vi "Test CSPD.vi"() -> ()   [LabVIEW 2020]
uses:
  epl-vi-lib/Signal Synthesis VIs/4th Generation/Classes/Level/LevelUnits.ctl
  epl-vi-lib/Signal Synthesis VIs/4th Generation/Classes/Filter/Shape.ctl
  epl-vi-lib/Signal Synthesis VIs/4th Generation/Classes/Filter/Units.ctl
  epl-vi-lib/Signal Synthesis VIs/4th Generation/Classes/Filter/Class.ctl
  epl-vi-lib/Signal Synthesis VIs/4th Generation/Classes/Level/Level.lvclass/Level.ctl
  epl-vi-lib/Signal Synthesis VIs/4th Generation/Classes/Filter/Filter.lvclass/Filter.ctl
  epl-vi-lib/Signal Synthesis VIs/4th Generation/Classes/Channel/Channel.lvclass/Channel.ctl
  epl-vi-lib/Signal Synthesis VIs/4th Generation/Classes/Waveforms/Noise/Noise.lvclass/Noise.ctl
  3524247a-8ae7-46d9-b71a-c66d4844bc9f.vi
  515af87e-e52d-4374-9cab-fcd7ae8fdb32.vi
  d0648034-2dec-4c64-9990-624be246044c.vi
  <vilib>/Analysis/baseanly.llb/Mean (DBL).vi
  6fae71c9-6d50-4778-9b27-4de804f51e00.vi
  <vilib>/Analysis/2dsp.llb/Cross Power (DBL).vi
  726719d0-53ab-4cde-bbae-18d33152857b.vi
  2604dc13-bcb2-40bf-816d-3a5cc3b7061b.vi
  1f3778f6-1701-4067-84f0-78bcc854d358.vi
  98786886-4506-48be-a372-97a999c07828.vi
  42c39028-ae27-4509-9454-5f7b85e5a68c.vi
  b4e7675a-24cb-4713-9642-d50581707a3a.vi
  epl-vi-lib/Signal Synthesis VIs/4th Generation/Classes/Waveforms/Noise/Write Weights.vi
  epl-vi-lib/Signal Synthesis VIs/4th Generation/Classes/Level/Write Units.vi
  epl-vi-lib/Signal Synthesis VIs/4th Generation/Classes/Level/Write Level.vi
  epl-vi-lib/Signal Synthesis VIs/4th Generation/Classes/Filter/Write Type.vi
  epl-vi-lib/Signal Synthesis VIs/4th Generation/Classes/Filter/Write Units.vi
  epl-vi-lib/Signal Synthesis VIs/4th Generation/Classes/Filter/Write BW (kHz).vi
  epl-vi-lib/Signal Synthesis VIs/4th Generation/Classes/Filter/Write CF (kHz).vi
  epl-vi-lib/Signal Synthesis VIs/4th Generation/Classes/Filter/Write Class.vi
  epl-vi-lib/Signal Synthesis VIs/4th Generation/Classes/Channel/Write Waveform.vi
  epl-vi-lib/Signal Synthesis VIs/4th Generation/Classes/Channel/Write Level.vi
  epl-vi-lib/Signal Synthesis VIs/4th Generation/Classes/Channel/Write Destination.vi
  epl-vi-lib/Signal Synthesis VIs/4th Generation/Classes/Channel/Write Filter.vi
  epl-vi-lib/Signal Synthesis VIs/4th Generation/Classes/Waveforms/Noise/Noise.lvclass
  D:/Development/epl-vi-lib/Signal Synthesis VIs/4th Generation/Classes/Waveforms/Waveform/Waveform.lvclass
  epl-vi-lib/Utility VIs/Math VIs/FFT x(t) to dB,Degrees (1D).vi
  epl-vi-lib/Signal Synthesis VIs/4th Generation/Classes/Channel/Channel.lvclass
  epl-vi-lib/Signal Synthesis VIs/4th Generation/Classes/Level/Level.lvclass
  epl-vi-lib/Signal Synthesis VIs/4th Generation/Classes/SignalManager/SignalManager.lvclass
  epl-vi-lib/Signal Synthesis VIs/4th Generation/Classes/Filter/Filter.lvclass
  <vilib>/Analysis/NI_AALPro.lvlib
  <vilib>/Analysis/NI_AALBase.lvlib
panel:
  out "Pcs 3":dbl
  out "mean":dbl format="%.7f"
  out "Pcs 2":dbl
  out "Pcs":dbl
  out "Px":dbl
  out "XY Graph":T1(graph)
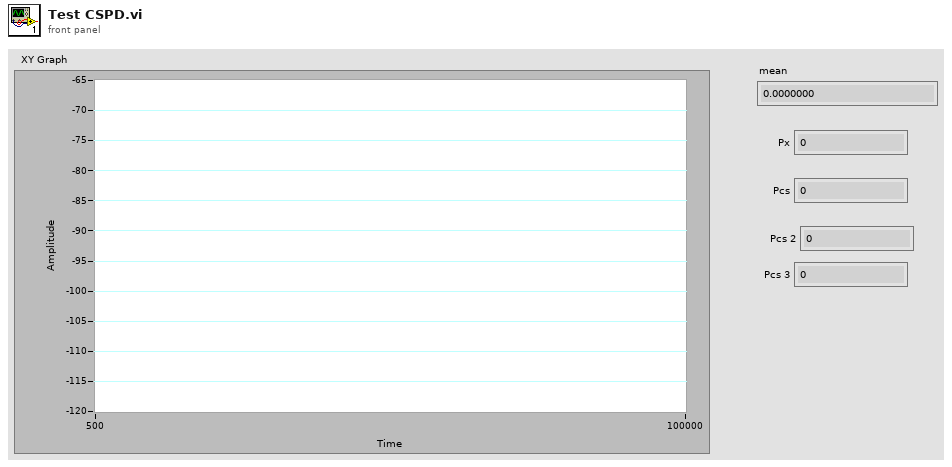
[diagram p1: front panel]
types:
  T1 = cluster{"Freq (Hz)":dbl[], "+Freq. Mag of FFT (dB rms)":dbl[]}[]
  T2 = typedef "Filter.lvclass/Class.ctl" = enum16{"Elliptic", "Butterworth", "Brickwall"}
  T3 = typedef "Filter.lvclass/Units.ctl" = enum16{"Linear", "Octaves", "Min-Max"}
  T4 = typedef "Filter.lvclass/Shape.ctl" = enum16{"OFF", "Lowpass", "Highpass", "Bandpass", "Bandstop"}
  T5 = typedef "Level.lvclass/LevelUnits.ctl" = enum16{"dB atten", "dB SPL", "dB Vrms", "Volts", "dB mW", "mW", "dB HL", "dB SL"}
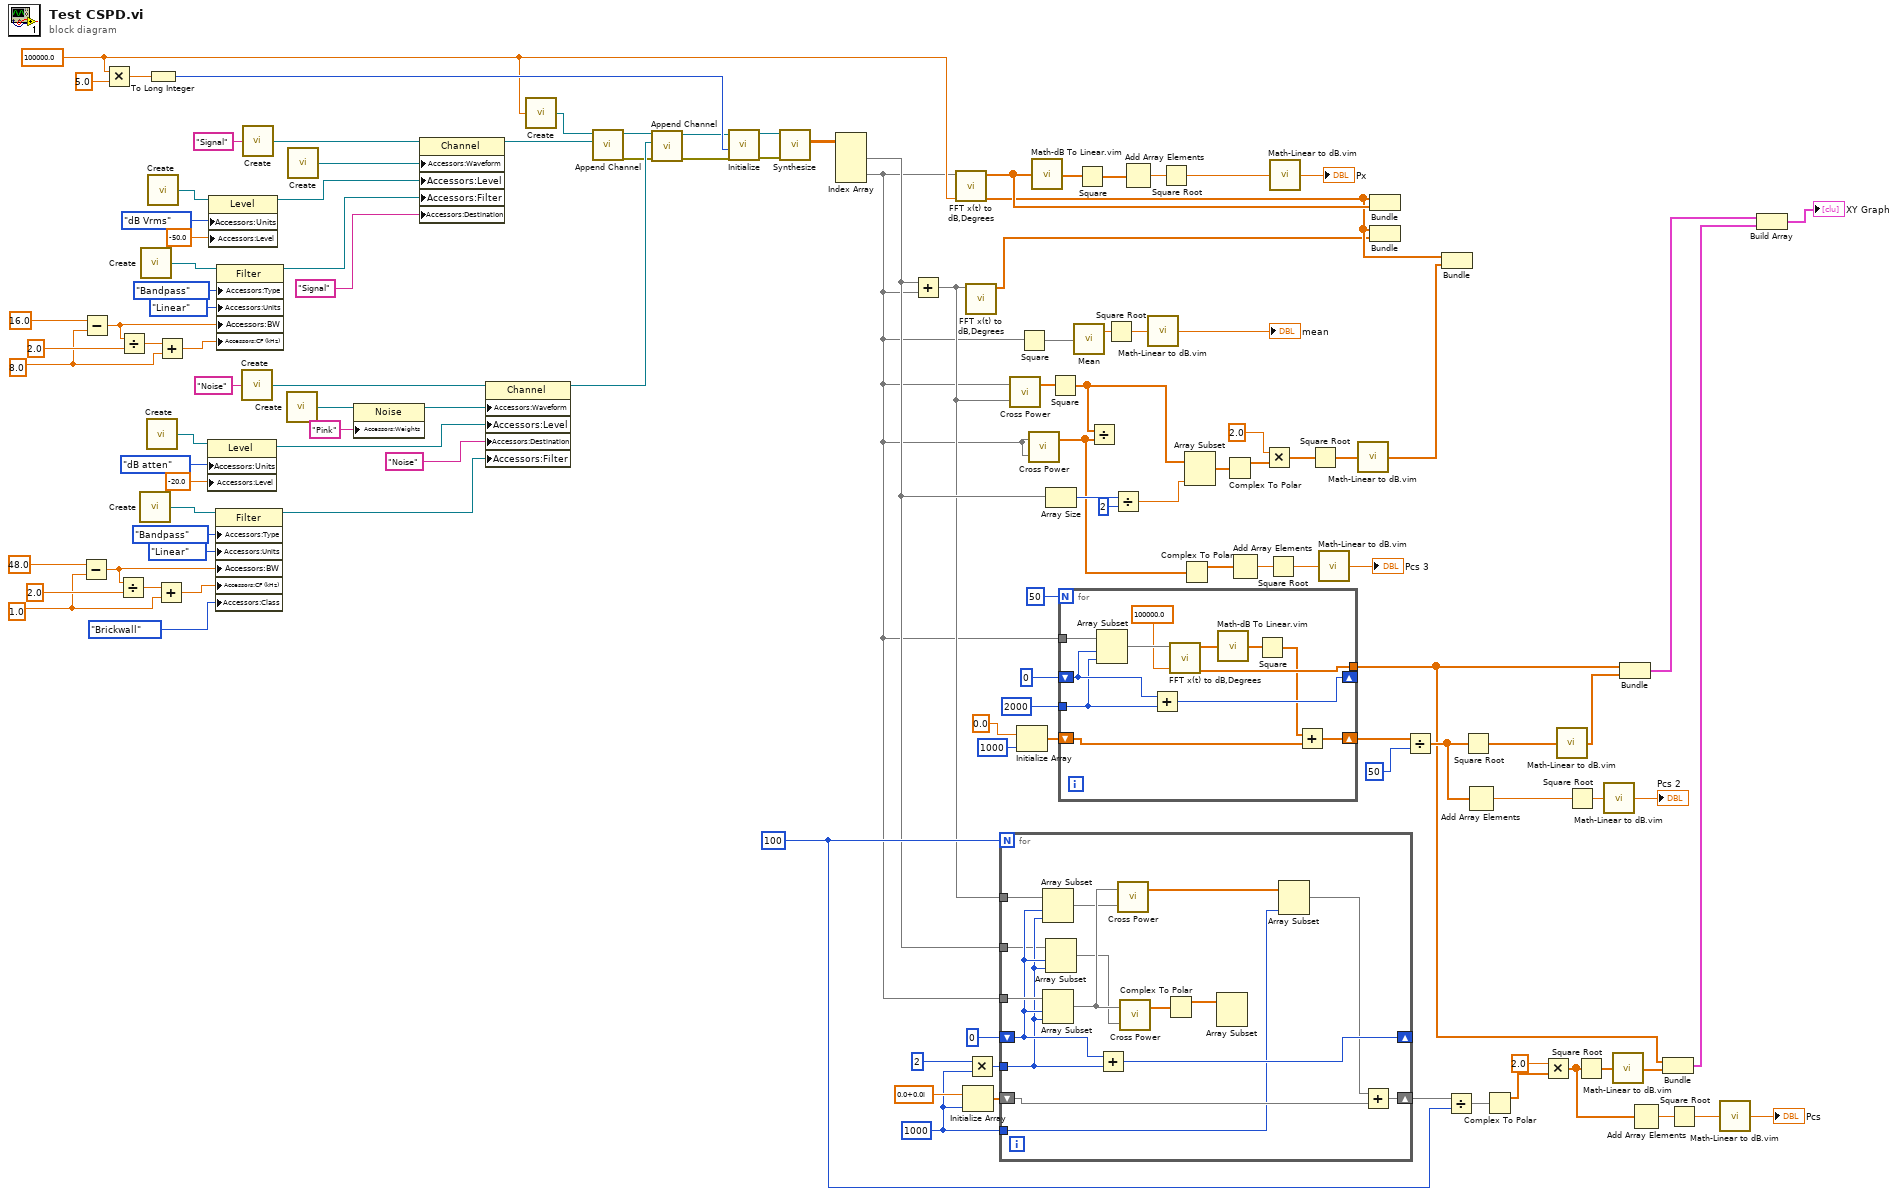
[diagram p0: block diagram]
diagram:
  w31 = 1000 ("dimension size")
  w29 = 100
  w81 = 1.0 ("High cutoff (kHz)")
  w97 = 100000.0 ("Fs (Hz)")
  w101 = 8.0 ("High cutoff (kHz)")
  n1 = Subtract(x=48.0 ("High cutoff (kHz)"), y=w81) -> (x-y=w85:dbl)
  n2 = Subtract(x=16.0 ("High cutoff (kHz)"), y=w101) -> (x-y=w108:dbl)
  n3 = Multiply(x=w97, y=5.0) -> (x*y=w99:dbl)
  n4 = Divide(x=w85, y=2.0) -> (x/y=w95:dbl)
  n5 = Divide(x=w108, y=2.0) -> (x/y=w118:dbl)
  n6 = call "Create.vi"() -> ("Filter"=w88:refnum<class "Filter.lvclass">)  [unwired: 15 in]
  n7 = call "Create.vi"() -> ("Filter"=w111:refnum<class "Filter.lvclass">)  [unwired: 15 in]
  n8 = call "Create.vi"() -> ("Level"=w92:refnum<class "Level.lvclass">)  [unwired: 15 in]
  n9 = To Long Integer(number=w99) -> (32bit integer=w98:i32)
  n10 = call "Create.vi"() -> ("Level"=w115:refnum<class "Level.lvclass">)  [unwired: 15 in]
  n11 = Add(x=w95, y=w81) -> (x+y=w84:dbl)
  n12 = Add(x=w118, y=w101) -> (x+y=w107:dbl)
  n13 = property class="Level"(reference=w92, "Accessors:Units"=LevelUnits."dB atten" ("Units"), "Accessors:Level"=-20.0 ("Level")) -> (reference out=w89:refnum<class "Level.lvclass">)  [unwired: 1 in, 1 out]
  n14 = property class="Level"(reference=w115, "Accessors:Units"=LevelUnits."dB Vrms" ("Units"), "Accessors:Level"=-50.0 ("Level")) -> (reference out=w112:refnum<class "Level.lvclass">)  [unwired: 1 in, 1 out]
  n15 = property class="Filter"(reference=w88, "Accessors:Type"=Shape."Bandpass" ("Type"), "Accessors:Units"=Units."Linear" ("Units"), "Accessors:BW"=w85, "Accessors:CF (kHz)"=w84, "Accessors:Class"=Class."Brickwall" ("Class")) -> (reference out=w9:refnum<class "Filter.lvclass">)  [unwired: 1 in, 1 out]
  n16 = property class="Filter"(reference=w111, "Accessors:Type"=Shape."Bandpass" ("Type"), "Accessors:Units"=Units."Linear" ("Units"), "Accessors:BW"=w108, "Accessors:CF (kHz)"=w107) -> (reference out=w106:refnum<class "Filter.lvclass">)  [unwired: 1 in, 1 out]
  n17 = call "Create.vi"("Name"="Noise") -> ("Channel"=w93:refnum<class "Channel.lvclass">)  [unwired: 14 in]
  n18 = call "Create.vi"("Name"="Signal") -> ("Channel"=w116:refnum<class "Channel.lvclass">)  [unwired: 14 in]
  n19 = call "Create.vi"() -> ("Noise"=w80:refnum<class "Noise.lvclass">)  [unwired: 15 in]
  n20 = call "Create.vi"() -> ("Noise"=w10:refnum<class "Noise.lvclass">)  [unwired: 15 in]
  n21 = property class="Noise"(reference=w80, "Accessors:Weights"="Pink" ("Weights")) -> (reference out=w79:refnum<class "Noise.lvclass">)  [unwired: 1 in, 1 out]
  n22 = property class="Channel"(reference=w116, "Accessors:Waveform"=w10, "Accessors:Level"=w112, "Accessors:Filter"=w106, "Accessors:Destination"="Signal") -> (reference out=w104:refnum<class "Channel.lvclass">)  [unwired: 1 in, 1 out]
  n23 = property class="Channel"(reference=w93, "Accessors:Waveform"=w79, "Accessors:Level"=w89, "Accessors:Destination"="Noise", "Accessors:Filter"=w9) -> (reference out=w76:refnum<class "Channel.lvclass">)  [unwired: 1 in, 1 out]
  n24 = call "Create.vi"("Fs (Hz)"=w97) -> ("SigMan"=w105:refnum<class "SignalManager.lvclass">)  [unwired: 14 in]
  n25 = call "Append Channel.vi"("Channel"=w104, "SignalManager in"=w105) -> ("error out"=w75:errorcluster, "SignalManager out"=w77:refnum<class "SignalManager.lvclass">)  [unwired: 8 in]
  n26 = call "Append Channel.vi"("error in (no error)"=w75, "Channel"=w76, "SignalManager in"=w77) -> ("error out"=w73:errorcluster, "SignalManager out"=w74:refnum<class "SignalManager.lvclass">)  [unwired: 7 in]
  n27 = call "Initialize.vi"("error in (no error)"=w73, "Npts"=w98, "SigMan in"=w74) -> ("error out"=w71:errorcluster, "SigMan out"=w72:refnum<class "SignalManager.lvclass">)  [unwired: 7 in]
  n28 = call "Synthesize.vi"("error in (no error)"=w71, "SigMan in"=w72) -> ("Array"=w70:dbl[][])  [unwired: 7 in, 2 out]
  n29 = Index Array(array=w70) -> (element #1=w5:dbl[], element #2=w2:dbl[])  [unwired: 4 in]
  n30 = Add(x=w5, y=w2) -> (x+y=w4:dbl[])
  n31 = call-poly "FFT x(t) to dB,Degrees.vi"("Fs (Hz)"=w97, "X"=w2) -> ("Freq (Hz)"=w52:dbl[], "+Freq. Mag of FFT (dB rms)"=w54:dbl[])  [unwired: 7 in, 1 out]
  n32 = Initialize Array(cdb 0.0+0.0i, w31) -> (w37:cdb[])
  n33 = call-poly "FFT x(t) to dB,Degrees.vi"("X"=w4) -> ("+Freq. Mag of FFT (dB rms)"=w19:dbl[])  [unwired: 8 in, 2 out]
  n34 = Multiply(x=2, y=w31) -> (x*y=w32:i32)
  n35 = for {
    N: w29 -> [_]
    tunnel: w2 -> [w135]
    shift-right: [w134] -> _
    shift-left: 0 -> [w126]
    tunnel: w32 -> [w125]
    shift-right: [w133] -> w36
    shift-left: w37 -> [w132]
    tunnel: w4 -> [w131]
    tunnel: w31 -> [w127]
    tunnel: w5 -> [w124]
    n36 = Array Subset(array=w131, index=w126, length=w125) -> (w128:dbl[])
    n37 = Array Subset(array=w135, index=w126, length=w125) -> (w129:dbl[])
    n38 = Array Subset(array=w124, index=w126, length=w125) -> (w123:dbl[])
    n39 = Add(x=w126, y=w125) -> (x+y=w134:i32)
    n40 = call-poly <vilib>:"Cross Power.vi"("Y"=w128, "X"=w129) -> ("Sxy"=w120:cdb[])  [unwired: 1 out]
    n41 = call-poly <vilib>:"Cross Power.vi"("Y"=w123, "X"=w129) -> ("Sxy"=w121:cdb[])  [unwired: 1 out]
    n42 = Complex To Polar(r * e^(i*theta)=w121) -> (r=w122:dbl[])  [unwired: 1 out]
    n43 = Array Subset(array=w122) -> ()  [unwired: 2 in, 1 out]
    n44 = Array Subset(array=w120, length=w127) -> (w130:cdb[])  [unwired: 1 in]
    n45 = Add(x=w130, y=w132) -> (x+y=w133:cdb[])
  }
  n46 = call-poly <vilib>:"Cross Power.vi"("Y"=w4, "X"=w2) -> ("Sxy"=w53:cdb[])  [unwired: 1 out]
  n47 = Initialize Array(0.0, 1000 ("dimension size")) -> (w45:dbl[])
  n48 = Square(x=w2) -> (x^2=w28:dbl[])
  n49 = call-poly <vilib>:"Cross Power.vi"("Y"=w2, "X"=w2) -> ("Sxy"=w17:cdb[])  [unwired: 1 out]
  n50 = call "Math-dB To Linear.vim"("dB"=w54) -> ("linear"=w66:dbl[])
  n51 = Array Size(array=w5) -> (size(s)=w62:i32)
  n52 = Square(x=w53) -> (x^2=w15:cdb[])
  n53 = for {
    N: 50 -> [_]
    tunnel: w2 -> [w147]
    shift-right: [w141] -> _
    shift-left: 0 -> [w143]
    tunnel: 2000 -> [w142]
    shift-right: [w140] -> w44
    shift-left: w45 -> [w139]
    tunnel: [w138] -> w6
    n54 = Array Subset(array=w147, index=w143, length=w142) -> (w146:dbl[])
    n55 = Add(x=w143, y=w142) -> (x+y=w141:i32)
    n56 = call-poly "FFT x(t) to dB,Degrees.vi"("Fs (Hz)"=100000.0, "X"=w146) -> ("Freq (Hz)"=w138:dbl[], "+Freq. Mag of FFT (dB rms)"=w144:dbl[])  [unwired: 7 in, 1 out]
    n57 = call "Math-dB To Linear.vim"("dB"=w144) -> ("linear"=w137:dbl[])
    n58 = Square(x=w137) -> (x^2=w136:dbl[])
    n59 = Add(x=w136, y=w139) -> (x+y=w140:dbl[])
  }
  n60 = call-poly <vilib>:"Mean.vi"("X"=w28) -> ("mean"=w27:dbl)  [unwired: 1 out]
  n61 = Square(x=w66) -> (x^2=w65:dbl[])
  n62 = Divide(x=w15, y=w17) -> ()  [unwired: 1 out]
  n63 = Square Root(x=w27) -> (sqrt(x)=w20:dbl)
  n64 = Divide(x=w62, y=2) -> (x/y=w60:dbl)
  n65 = Add Array Elements(numeric array=w65) -> (sum=w69:dbl)
  n66 = call "Math-Linear to dB.vim"("linear"=w20) -> ("dB"=→"mean":dbl)
  n67 = Square Root(x=w69) -> (sqrt(x)=w67:dbl)
  n68 = Complex To Polar(r * e^(i*theta)=w17) -> (r=w21:dbl[])  [unwired: 1 out]
  n69 = Array Subset(array=w15, length=w60) -> (w61:cdb[])  [unwired: 1 in]
  n70 = Complex To Polar(r * e^(i*theta)=w61) -> (r=w55:dbl[])  [unwired: 1 out]
  n71 = Add Array Elements(numeric array=w21) -> (sum=w24:dbl)
  n72 = Multiply(x=2.0, y=w55) -> (x*y=w25:dbl[])
  n73 = Square Root(x=w24) -> (sqrt(x)=w22:dbl)
  n74 = call "Math-Linear to dB.vim"("linear"=w67) -> ("dB"=→"Px":dbl)
  n75 = Square Root(x=w25) -> (sqrt(x)=w18:dbl[])
  n76 = call "Math-Linear to dB.vim"("linear"=w22) -> ("dB"=→"Pcs 3":dbl)
  n77 = call "Math-Linear to dB.vim"("linear"=w18) -> ("dB"=w51:dbl[])
  n78 = Bundle("Freq (Hz)"=w52, "+Freq. Mag of FFT (dB rms)"=w54) -> ()  [unwired: 1 in, 1 out]
  n79 = Bundle("Freq (Hz)"=w52, "+Freq. Mag of FFT (dB rms)"=w19) -> ()  [unwired: 1 in, 1 out]
  n80 = Divide(x=w44, y=50) -> (x/y=w11:dbl[])
  n81 = Bundle("Freq (Hz)"=w52, "dB"=w51) -> ()  [unwired: 1 in, 1 out]
  n82 = Divide(x=w36, y=w29) -> (x/y=w34:cdb[])
  n83 = Square Root(x=w11) -> (sqrt(x)=w12:dbl[])
  n84 = Add Array Elements(numeric array=w11) -> (sum=w42:dbl)
  n85 = Complex To Polar(r * e^(i*theta)=w34) -> (r=w3:dbl[])  [unwired: 1 out]
  n86 = Multiply(x=2.0, y=w3) -> (x*y=w1:dbl[])
  n87 = call "Math-Linear to dB.vim"("linear"=w12) -> ("dB"=w8:dbl[])
  n88 = Square Root(x=w42) -> (sqrt(x)=w40:dbl)
  n89 = Square Root(x=w1) -> (sqrt(x)=w35:dbl[])
  n90 = call "Math-Linear to dB.vim"("linear"=w40) -> ("dB"=→"Pcs 2":dbl)
  n91 = call "Math-Linear to dB.vim"("linear"=w35) -> ("dB"=w7:dbl[])
  n92 = Bundle("Freq (Hz)"=w6, "dB"=w8) -> (w13:cluster{"Freq (Hz)":dbl[], "dB":dbl[]})  [unwired: 1 in]
  n93 = Add Array Elements(numeric array=w1) -> (sum=w58:dbl)
  n94 = Bundle("Freq (Hz)"=w6, "dB"=w7) -> (w14:cluster{"Freq (Hz)":dbl[], "dB":dbl[]})  [unwired: 1 in]
  n95 = Square Root(x=w58) -> (sqrt(x)=w56:dbl)
  n96 = call "Math-Linear to dB.vim"("linear"=w56) -> ("dB"=→"Pcs":dbl)
  n97 = Build Array(w13, w14) -> (→"XY Graph":cluster{"Freq (Hz)":dbl[], "dB":dbl[]}[])
